vi "aboutMsg.vi"(8 "error in (no error)":errorcluster, 11 "simonMessages in":refnum<class "simonMessages.lvclass">) -> (0 "error out":errorcluster, 3 "simonMessages out":refnum<class "simonMessages.lvclass">)   [LabVIEW 2019, in "simonMessages.lvclass"]
uses:
  simonMessages.lvclass
  simonMessages.lvclass/simonMessages.ctl
  TextDisplay/TextDisplay Class.lvclass
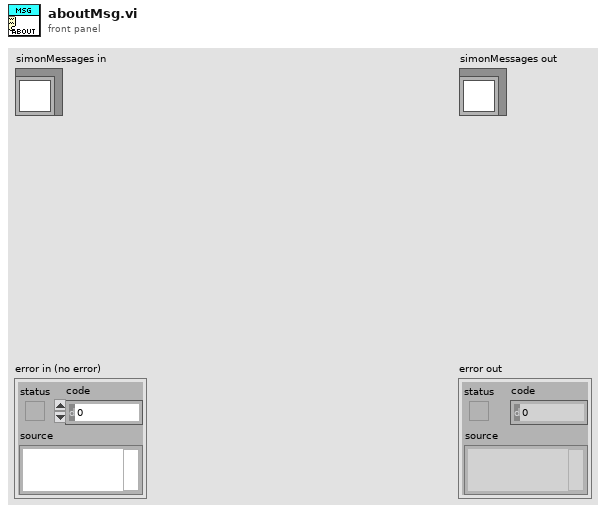
[diagram p1: front panel]
types:
  T1 = map{string, cluster{"Text":string, "Size":u8, "Justification":enum16{"Left", "Center", "Right"}, "Display Type":string}}
  T2 = cluster{"Text":string, "Size":u8, "Justification":enum16{"Left", "Center", "Right"}, "Display Type":string}
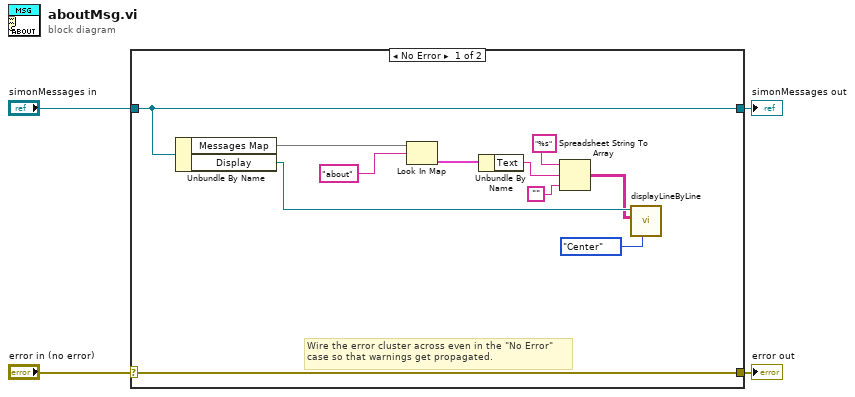
[diagram p0: block diagram]
diagram:
  n1 = case shown="No Error" "error in (no error)" {
    selector: "error in (no error)" -> [w15 w17]
    tunnel: [w15 w17] -> w3
    tunnel: [w14 w16] -> w1
    tunnel: "simonMessages in" -> [w14 w16]
    frame No Error {
      # "Wire the error cluster across even in the \"No Error\"\ncase so that warnings get propagated."
      n2 = Unbundle By Name(w14) -> ("Messages Map"=w13:T1, "Display"=w10:refnum<class "TextDisplay Class.lvclass">)
      n3 = Look In Map(map=w13, key="about") -> (value=w11:T2)  [unwired: 1 in, 1 out]
      n4 = Unbundle By Name(w11) -> ("Text"=w8:string)
      n5 = Spreadsheet String To Array(format string="%s", spreadsheet string=w8, array type (2D Dbl)="") -> (array=w9:string[][])  [unwired: 1 in]
      n6 = call "displayLineByLine.vi"("Justification"=enum16{"Left", "Center", "Right"}."Center", "scoreLog"=w9, "TextDisplay Class in"=w10) -> ()  [unwired: 7 in, 2 out]
    }
    frame Error {
    }
  }
  "error out" <- w3
  "simonMessages out" <- w1
